vi "SUMMER SUNDAY BYTE[8].vi"() -> ()   [LabVIEW 2009]
uses:
  <vilib>/ULx/Create Channel.llb/ULx Create Channel (AI-Voltage-Basic).vi
  <vilib>/ULx/Create Channel.llb/ULx Create Channel (DO-Digital Output).vi
  <vilib>/ULx/Create Channel.llb/ULx Create Channel (DI-Digital Input).vi
  <vilib>/ULx/Write.llb/ULx Write (Digital Bool 1Line 1Point).vi
  <vilib>/ULx/Read.llb/ULx Read (Analog DBL 1Chan 1Samp).vi
  <vilib>/ULx/Read.llb/ULx Read (Digital 1D U8 NChan 1Samp).vi
panel:
  out "max value":u8
  out "POWER":bool
  out "data":dbl format="%_6g"
  out "ENERGY LEVEL":dbl(knob) scale=0.0..15.0
  out "Beam Pot":dbl format="%_6g"
  out "READY 2":bool
  out "DUMP":bool
  out "POWER":bool
  out "?":bool
  out "?":bool
  out "?":bool
  out "?":bool
  out "?":bool
  out "?":bool
  out "?":bool
  out "?":bool
  out "?":bool
  out "?":bool
  out "OPEN":bool
  out "CLOSED":bool
  out "READY":bool
  out "FAULT":bool
  out "MAGNET FORCE":dbl(slide) scale=0.0..10.0
  out "READY":bool
  out "TEMPERATURE":dbl(slide) scale=0.0..100.0
  in  "stop":bool
  out "?":bool
  out "?":bool
  out "?":bool
  out "?":bool
  out "FAULT":bool
  out "POWER":bool
  out "FLOW IN GPM":dbl(knob) scale=0.0..15.0
  # "USERS LAB AREA"
  # "BEAM STATUS"
  # "ROOM"
  # "XRAY"
  # "PUMP STATION"
  # "MAGNET STATUS"
  # "ORBIT"
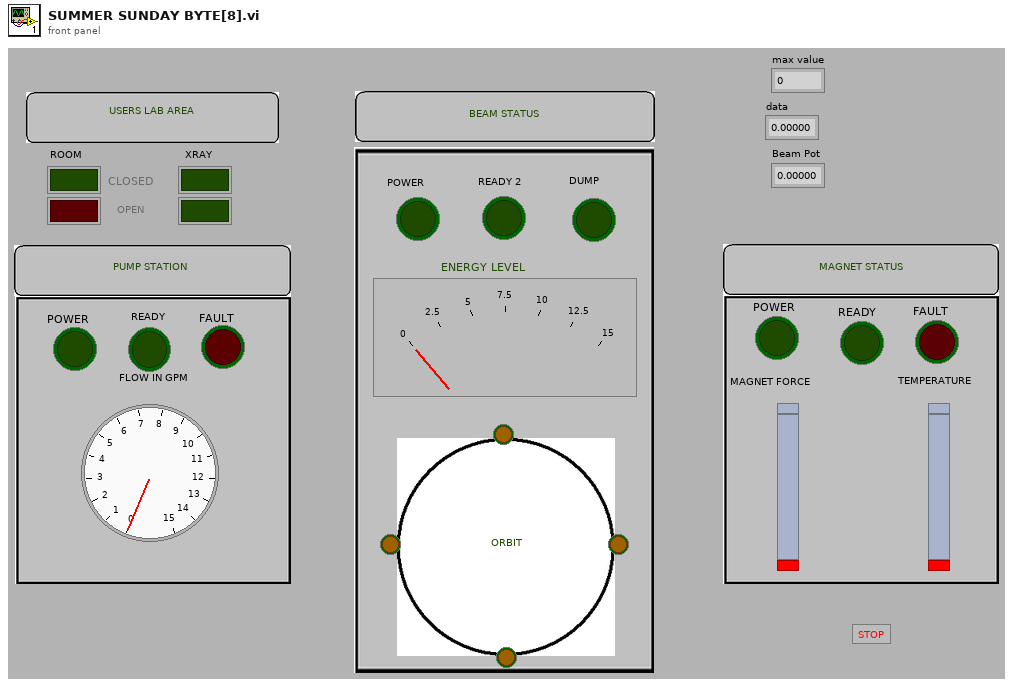
[diagram p1: front panel]
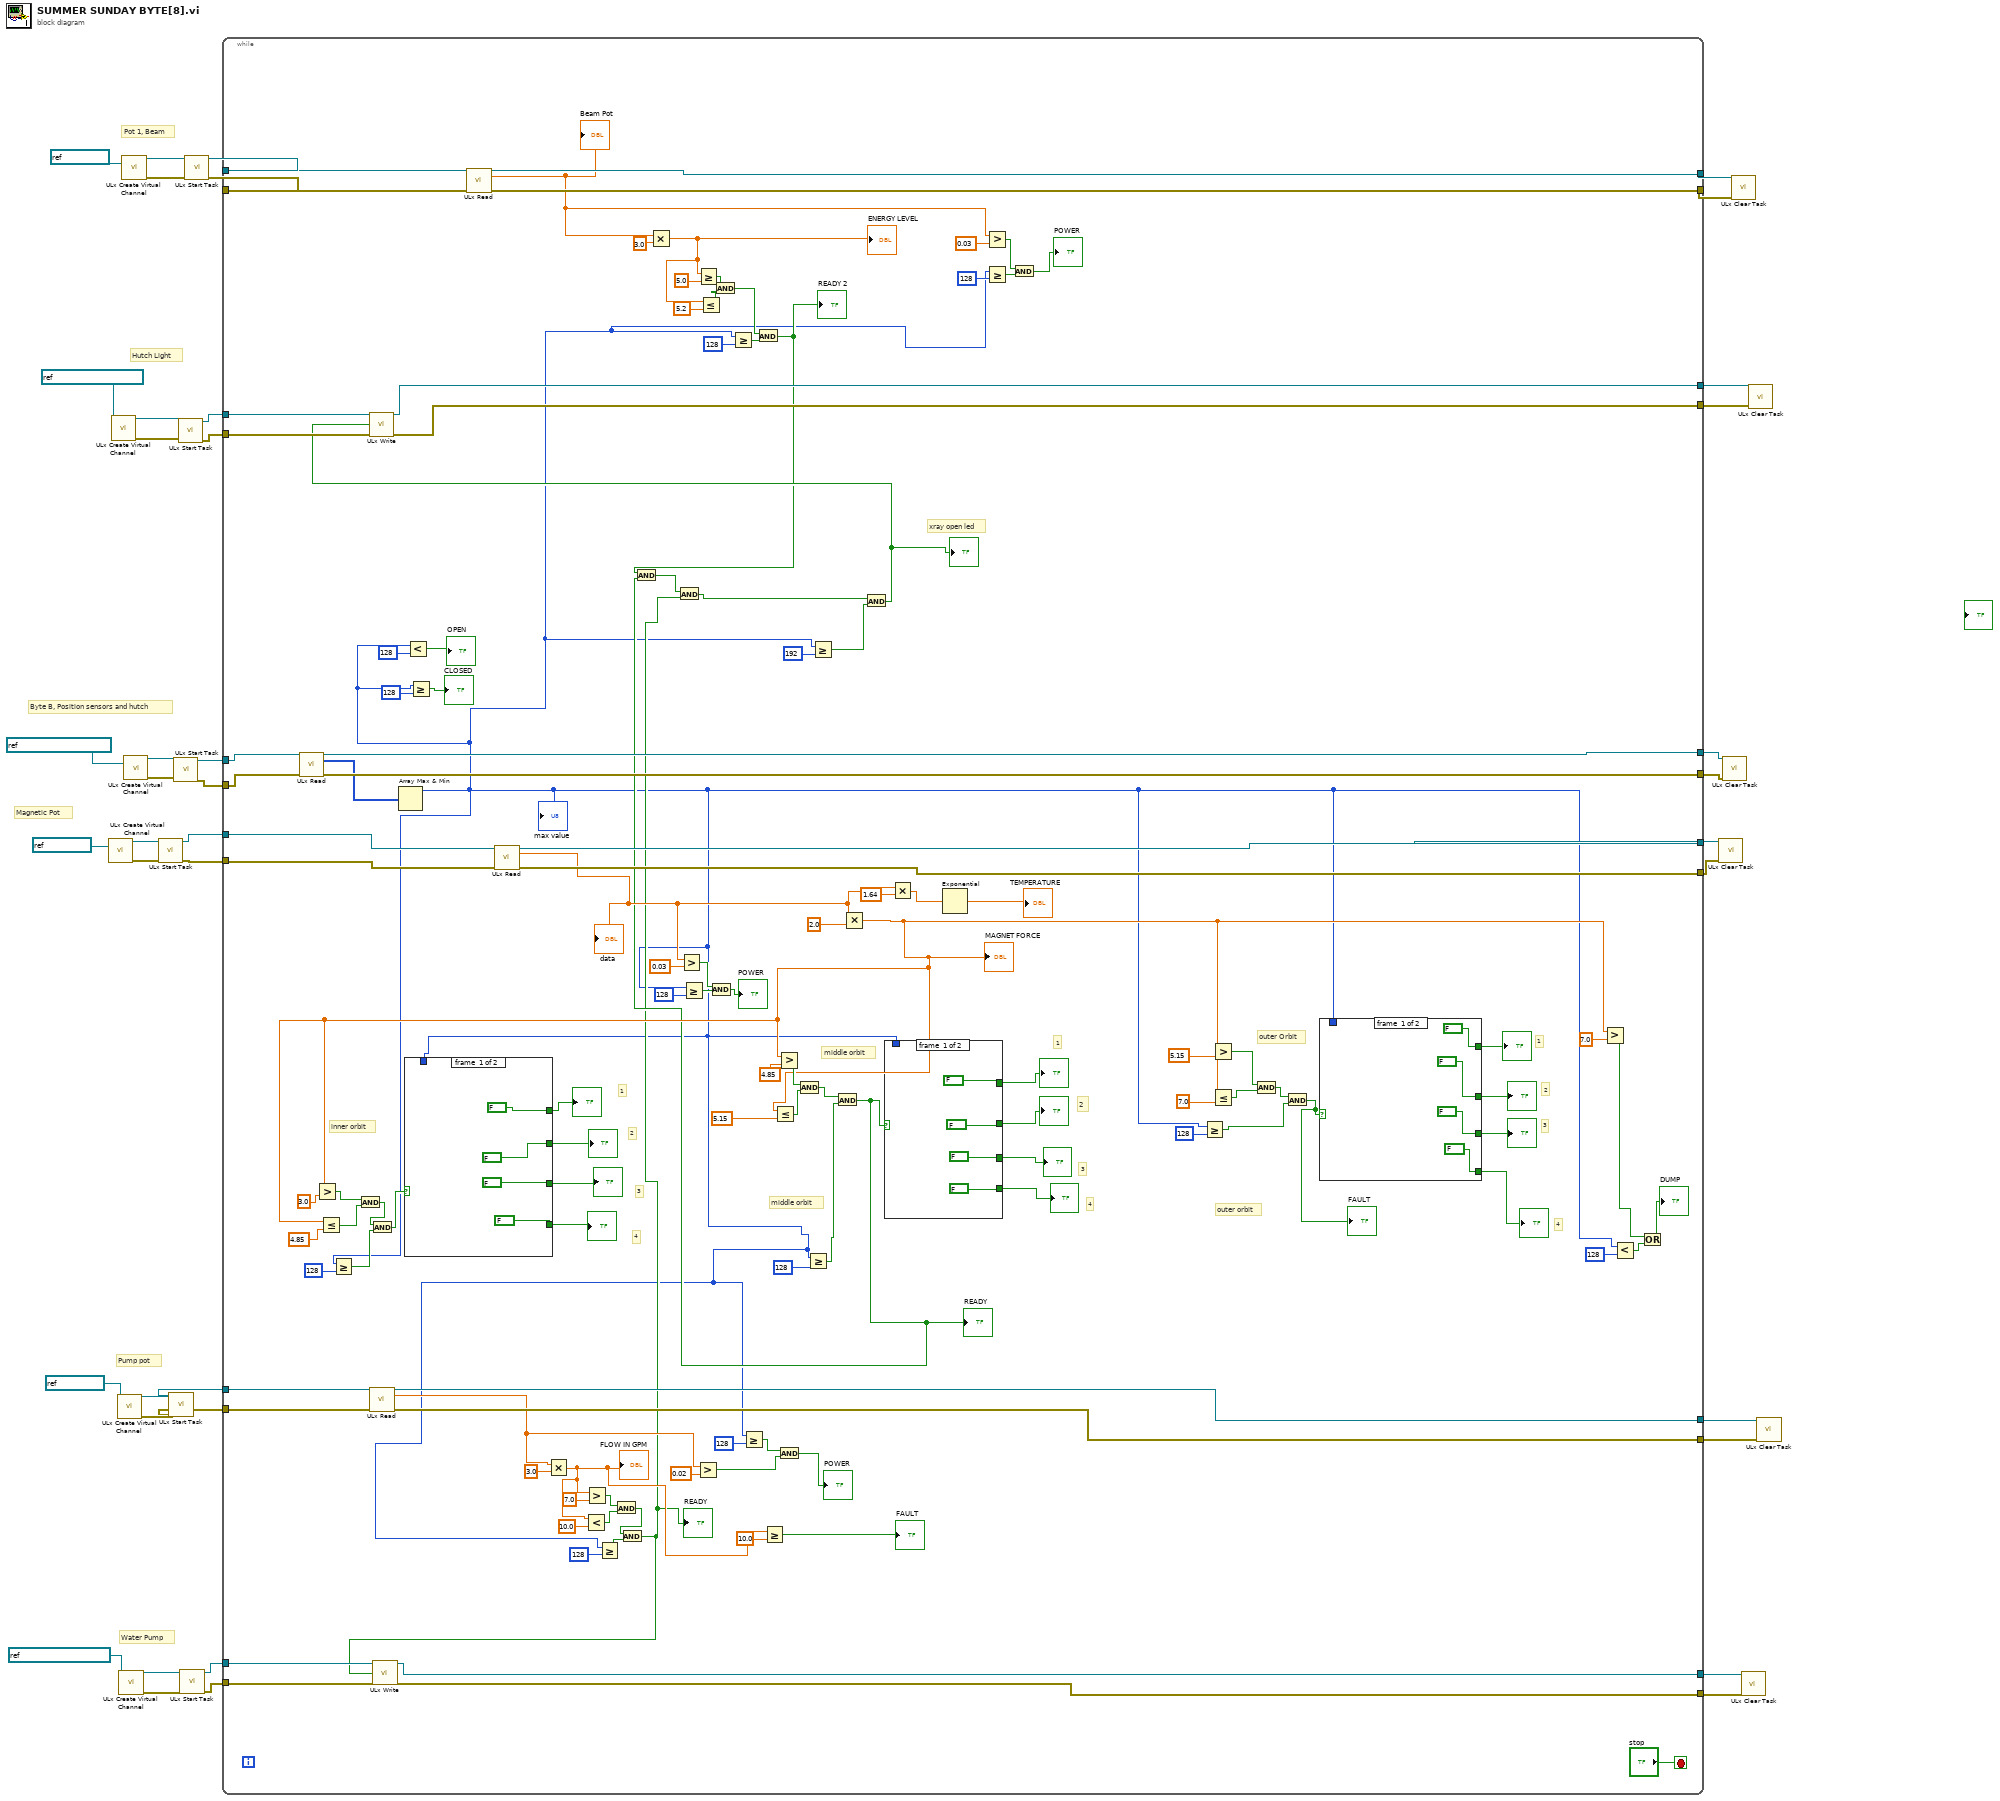
[diagram p0: block diagram]
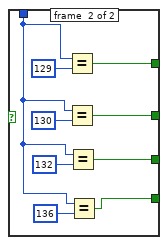
[diagram p2: hidden frame]
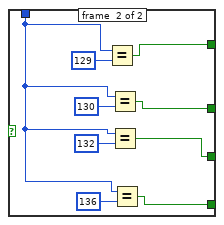
[diagram p3: hidden frame]
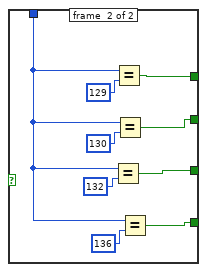
[diagram p4: hidden frame]
diagram:
  # "Water Pump"
  # "Pump pot"
  # "Hutch Light"
  # "Byte B, Position sensors and hutch"
  # "Magnetic Pot"
  # "Pot 1, Beam"
  n1 = call-poly <vilib>:"ULx Create Virtual Channel.vi"("physical channels"=refnum<k21> "Dev0/Ai1") -> ("task out"=w36:refnum<k24>, "error out"=w35:errorcluster)  [unwired: 13 in]
  n2 = call-poly <vilib>:"ULx Create Virtual Channel.vi"("lines"=refnum<k21> "Dev0/1stPortA/Do0") -> ("task out"=w21:refnum<k24>, "error out"=w20:errorcluster)  [unwired: 13 in]
  n3 = call-poly <vilib>:"ULx Create Virtual Channel.vi"("physical channels"=refnum<k21> "Dev0/Ai2") -> ("task out"=w28:refnum<k24>, "error out"=w27:errorcluster)  [unwired: 13 in]
  n4 = call-poly <vilib>:"ULx Create Virtual Channel.vi"("lines"=refnum<k21> "Dev0/1stPortA/Do1") -> ("task out"=w7:refnum<k24>, "error out"=w6:errorcluster)  [unwired: 13 in]
  n5 = call-poly <vilib>:"ULx Create Virtual Channel.vi"("physical channels"=refnum<k21> "Dev0/Ai0") -> ("task out"=w42:refnum<k24>, "error out"=w41:errorcluster)  [unwired: 13 in]
  n6 = call-poly <vilib>:"ULx Create Virtual Channel.vi"("lines"=refnum<k21> "Dev0/1stPortB/Di0:7") -> ("task out"=w14:refnum<k24>, "error out"=w13:errorcluster)  [unwired: 13 in]
  n7 = call <vilib>:"ULx Start Task.vi"("task in"=w36, "error in"=w35) -> ("task out"=w34:refnum<k24>, "error out"=w33:errorcluster)  [unwired: 12 in]
  n8 = call <vilib>:"ULx Start Task.vi"("task in"=w28, "error in"=w27) -> ("task out"=w26:refnum<k24>, "error out"=w25:errorcluster)  [unwired: 12 in]
  n9 = call <vilib>:"ULx Start Task.vi"("task in"=w14, "error in"=w13) -> ("task out"=w12:refnum<k24>, "error out"=w11:errorcluster)  [unwired: 12 in]
  n10 = call <vilib>:"ULx Start Task.vi"("task in"=w21, "error in"=w20) -> ("task out"=w18:refnum<k24>, "error out"=w17:errorcluster)  [unwired: 12 in]
  n11 = call <vilib>:"ULx Start Task.vi"("task in"=w7, "error in"=w6) -> ("task out"=w5:refnum<k24>, "error out"=w4:errorcluster)  [unwired: 12 in]
  n12 = call <vilib>:"ULx Start Task.vi"("task in"=w42, "error in"=w41) -> ("task out"=w40:refnum<k24>, "error out"=w39:errorcluster)  [unwired: 12 in]
  n13 = while {
    tunnel: w40 -> [w163]
    tunnel: w39 -> [w162]
    tunnel: [w161] -> w38
    tunnel: [w160] -> w37
    tunnel: w34 -> [w158]
    tunnel: w33 -> [w157]
    tunnel: [w156] -> w32
    tunnel: [w155] -> w31
    tunnel: w26 -> [w117]
    tunnel: w25 -> [w116]
    tunnel: [w115] -> w23
    tunnel: [w114] -> w22
    tunnel: w18 -> [w88]
    tunnel: w17 -> [w87]
    tunnel: [w86] -> w16
    tunnel: [w85] -> w15
    tunnel: w12 -> [w84]
    tunnel: w11 -> [w83]
    tunnel: [w82] -> w9
    tunnel: [w81] -> w8
    tunnel: w5 -> [w54]
    tunnel: w4 -> [w53]
    tunnel: [w52] -> w3
    tunnel: [w51] -> w2
    stop <- "stop" stop-if-true
    # "xray open led"
    # "outer Orbit"
    # "middle orbit"
    # "4"
    # "3"
    # "2"
    # "1"
    # "1"
    # "2"
    # "3"
    # "4"
    # "4"
    # "3"
    # "2"
    # "1"
    # "outer orbit"
    # "inner orbit"
    # "middle orbit"
    n14 = call-poly <vilib>:"ULx Read.vi"("task in"=w84, "error in"=w83) -> ("task out"=w82:refnum<k24>, "data"=w80:u8[], "error out"=w81:errorcluster)  [unwired: 11 in]
    n15 = call-poly <vilib>:"ULx Read.vi"("task in"=w117, "error in"=w116) -> ("task out"=w115:refnum<k24>, "data"=w110:dbl, "error out"=w114:errorcluster)  [unwired: 11 in]
    n16 = Array Max & Min(array=w80) -> (max value=w44:u8)  [unwired: 3 out]
    "max value" <- w44
    n17 = Greater Or Equal?(x=w44, y=i16 128) -> (x >= y?=w142:bool)
    n18 = Less?(x=w44, y=u8 128) -> (x < y?=→"OPEN":bool)
    n19 = Greater Or Equal?(x=w44, y=u8 128) -> (x >= y?=→"CLOSED":bool)
    n20 = call-poly <vilib>:"ULx Read.vi"("task in"=w163, "error in"=w162) -> ("task out"=w161:refnum<k24>, "data"=w89:dbl, "error out"=w160:errorcluster)  [unwired: 11 in]
    "Beam Pot" <- w89
    n21 = call-poly <vilib>:"ULx Read.vi"("task in"=w158, "error in"=w157) -> ("task out"=w156:refnum<k24>, "data"=w93:dbl, "error out"=w155:errorcluster)  [unwired: 11 in]
    "data" <- w93
    n22 = Multiply(x=w110, y=3.0) -> (x*y=w99:dbl)
    "FLOW IN GPM" <- w99
    n23 = Less?(x=w99, y=10.0) -> (x < y?=w97:bool)
    n24 = Greater?(x=w99, y=7.0) -> (0:w98:bool)
    n25 = Greater Or Equal?(x=w44, y=u8 128) -> (x >= y?=w69:bool)
    n26 = And(x=w98, y=w97) -> (x .and. y?=w67:bool)
    n27 = And(x=w67, y=w69) -> (x .and. y?=w45:bool)
    "READY" <- w45
    n28 = call-poly <vilib>:"ULx Write.vi"("task in"=w54, "data"=w45, "error in"=w53) -> ("task out"=w52:refnum<k24>, "error out"=w51:errorcluster)  [unwired: 10 in, 1 out]
    n29 = Multiply(x=w89, y=3.0) -> (x*y=w107:dbl)
    "ENERGY LEVEL" <- w107
    n30 = Greater?(x=w93, y=0.03) -> (0:w72:bool)
    n31 = Greater Or Equal?(x=w44, y=u8 128) -> (x >= y?=w71:bool)
    n32 = Greater?(x=w110, y=0.02) -> (0:w64:bool)
    n33 = Greater Or Equal?(x=w107, y=5.0) -> (x >= y?=w105:bool)
    n34 = Less Or Equal?(x=w107, y=5.2) -> (x <= y?=w104:bool)
    n35 = And(x=w72, y=w71) -> (x .and. y?=→"POWER":bool)
    n36 = And(x=w105, y=w104) -> (x .and. y?=w59:bool)
    n37 = Greater Or Equal?(x=w44, y=u8 128) -> (x >= y?=w61:bool)
    n38 = Greater Or Equal?(x=w44, y=u8 128) -> (x >= y?=w65:bool)
    n39 = And(x=w59, y=w61) -> (x .and. y?=w58:bool)
    "READY 2" <- w58
    n40 = Greater Or Equal?(x=w99, y=10.0) -> (x >= y?=→"FAULT":bool)
    n41 = And(x=w65, y=w64) -> (x .and. y?=→"POWER":bool)
    n42 = Greater Or Equal?(x=w44, y=i16 128) -> (x >= y?=w79:bool)
    n43 = Greater Or Equal?(x=w44, y=u8 192) -> (x >= y?=w74:bool)
    n44 = Multiply(x=w93, y=2.0) -> (x*y=w135:dbl)
    "MAGNET FORCE" <- w135
    n45 = Greater?(x=w135, y=3.0) -> (0:w151:bool)
    n46 = Less Or Equal?(x=w135, y=4.85) -> (x <= y?=w152:bool)
    n47 = And(x=w151, y=w152) -> (x .and. y?=w144:bool)
    n48 = And(x=w144, y=w142) -> (x .and. y?=w143:bool)
    n49 = case shown="True" w143 {
      tunnel: [FALSE w198] -> w120
      tunnel: [FALSE w197] -> w121
      tunnel: [FALSE w196] -> w118
      tunnel: [FALSE w195] -> w119
      tunnel: w44 -> [_ w203]
      frame #0 {
      }
      frame #1 {
        n50 = Equal?(x=w203, y=i16 132) -> (x = y?=w196:bool)
        n51 = Equal?(x=w203, y=i16 129) -> (x = y?=w198:bool)
        n52 = Equal?(x=w203, y=i16 130) -> (x = y?=w197:bool)
        n53 = Equal?(x=w203, y=i16 136) -> (x = y?=w195:bool)
      }
    }
    "?" <- w121
    "?" <- w118
    "?" <- w119
    "?" <- w120
    n54 = Less Or Equal?(x=w135, y=5.15) -> (x <= y?=w148:bool)
    n55 = Greater?(x=w135, y=4.85) -> (0:w149:bool)
    n56 = And(x=w149, y=w148) -> (x .and. y?=w141:bool)
    n57 = And(x=w141, y=w79) -> (x .and. y?=w77:bool)
    "READY" <- w77
    n58 = And(x=w58, y=w77) -> (x .and. y?=w76:bool)
    n59 = And(x=w76, y=w45) -> (x .and. y?=w75:bool)
    n60 = And(x=w75, y=w74) -> (x .and. y?=w73:bool)
    "?" <- w73
    n61 = call-poly <vilib>:"ULx Write.vi"("task in"=w88, "data"=w73, "error in"=w87) -> ("task out"=w86:refnum<k24>, "error out"=w85:errorcluster)  [unwired: 10 in, 1 out]
    n62 = case shown="True" w77 {
      tunnel: [FALSE w177] -> w130
      tunnel: [FALSE w176] -> w129
      tunnel: [FALSE w175] -> w128
      tunnel: [FALSE w174] -> w127
      tunnel: w44 -> [_ w173]
      frame #0 {
      }
      frame #1 {
        n63 = Equal?(x=w173, y=i16 129) -> (x = y?=w177:bool)
        n64 = Equal?(x=w173, y=i16 130) -> (x = y?=w176:bool)
        n65 = Equal?(x=w173, y=i16 132) -> (x = y?=w175:bool)
        n66 = Equal?(x=w173, y=i16 136) -> (x = y?=w174:bool)
      }
    }
    "?" <- w130
    "?" <- w129
    "?" <- w128
    "?" <- w127
    n67 = Multiply(x=w93, y=1.64) -> (x*y=w91:dbl)
    n68 = Exponential(1:w91) -> (0:→"TEMPERATURE":dbl)
    n69 = Greater?(x=w89, y=0.03) -> (0:w56:bool)
    n70 = Greater Or Equal?(x=w44, y=u8 128) -> (x >= y?=w62:bool)
    n71 = And(x=w56, y=w62) -> (x .and. y?=→"POWER":bool)
    n72 = Greater Or Equal?(x=w44, y=i16 128) -> (x >= y?=w125:bool)
    n73 = Greater?(x=w135, y=5.15) -> (0:w146:bool)
    n74 = Less Or Equal?(x=w135, y=7.0) -> (x <= y?=w145:bool)
    n75 = And(x=w146, y=w145) -> (x .and. y?=w134:bool)
    n76 = And(x=w134, y=w125) -> (x .and. y?=w94:bool)
    "FAULT" <- w94
    n77 = case shown="True" w94 {
      tunnel: [FALSE w182] -> w139
      tunnel: [FALSE w183] -> w138
      tunnel: [FALSE w184] -> w137
      tunnel: [FALSE w185] -> w136
      tunnel: w44 -> [_ w190]
      frame #0 {
      }
      frame #1 {
        n78 = Equal?(x=w190, y=i16 129) -> (x = y?=w185:bool)
        n79 = Equal?(x=w190, y=i16 130) -> (x = y?=w184:bool)
        n80 = Equal?(x=w190, y=i16 132) -> (x = y?=w183:bool)
        n81 = Equal?(x=w190, y=i16 136) -> (x = y?=w182:bool)
      }
    }
    "?" <- w136
    "?" <- w137
    "?" <- w138
    "?" <- w139
    n82 = Greater?(x=w135, y=7.0) -> (0:w95:bool)
    n83 = Less?(x=w44, y=i16 128) -> (x < y?=w122:bool)
    n84 = Or(x=w95, y=w122) -> (x .or. y?=→"DUMP":bool)
  }
  n85 = call <vilib>:"ULx Clear Task.vi"("task in"=w32, "error in"=w31) -> ()  [unwired: 13 in, 1 out]
  n86 = call <vilib>:"ULx Clear Task.vi"("task in"=w9, "error in"=w8) -> ()  [unwired: 13 in, 1 out]
  n87 = call <vilib>:"ULx Clear Task.vi"("task in"=w38, "error in"=w37) -> ()  [unwired: 13 in, 1 out]
  n88 = call <vilib>:"ULx Clear Task.vi"("task in"=w3, "error in"=w2) -> ()  [unwired: 13 in, 1 out]
  n89 = call <vilib>:"ULx Clear Task.vi"("task in"=w16, "error in"=w15) -> ()  [unwired: 13 in, 1 out]
  n90 = call <vilib>:"ULx Clear Task.vi"("task in"=w23, "error in"=w22) -> ()  [unwired: 13 in, 1 out]
